vi "Eval Condition.vi"(7 "Variables":refnum<class "Variables.lvclass">, 8 "error in (no error)":errorcluster, 9 "Sequence Time":T1, 11 "SeqRunning Condition in":refnum<class "SeqRunning Condition.lvclass">) -> (0 "error out":errorcluster, 2 "Result":bool, 3 "SeqRunning Condition out":refnum<class "SeqRunning Condition.lvclass">)   [LabVIEW 2020, in "VolatusSeq.lvlib" / "SeqRunning Condition.lvclass"]
uses:
  SeqRunning Condition.lvclass
  SeqRunning Condition.lvclass/SeqRunning Condition.ctl
  Volatus/MessageQ/MessageQ.lvclass
  Sequence Status Value/Sequence Status Value.lvclass
  Variables/Variables.lvclass
  Sequence Time.ctl
  VolatusSeq.lvlib
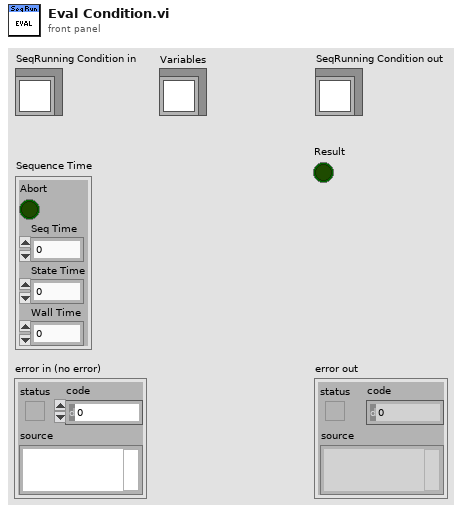
[diagram p1: front panel]
types:
  T1 = typedef "VolatusSeq.lvlib/Sequence Time.ctl" = cluster{"Abort":bool, "Seq Time":dbl, "State Time":dbl, "Wall Time":dbl}
  T2 = typedef "VolatusSeq.lvlib/Sequence Status.ctl" = cluster{"Name":string, "State":string, "Time":T1, "Running":bool, "Start Time":dbl, "Previous Duration":i64, "Previous Late":bool}
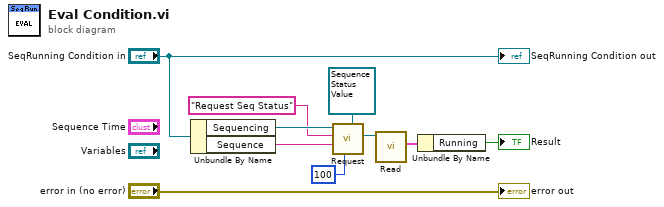
[diagram p0: block diagram]
diagram:
  n1 = Unbundle By Name("SeqRunning Condition in") -> ("Sequencing"=w9:refnum<class "MessageQ.lvclass">, "Sequence"=w7:string)
  n2 = call "Request.vi"("Response Type (None)"=refnum<class "Sequence Status Value.lvclass"> refnum ("VolatusSeq.lvlib:Sequence Status Value.lvclass"), "Timeout ms (1000)"=100, "Data"=w7, "ID"="Request Seq Status", "MessageQ in"=w9) -> ("Response"=w3:refnum<class "Sequence Status Value.lvclass">)  [unwired: 4 in, 2 out]
  n3 = call "Read.vi"("Sequence Status Value in"=w3) -> ("Sequence Status"=w2:T2)  [unwired: 10 in]
  n4 = Unbundle By Name(w2) -> ("Running"=→"Result":bool)
  "error out" <- "error in (no error)"
  "SeqRunning Condition out" <- "SeqRunning Condition in"
